vi "Set Path.vi"(8 "error in (no error)":errorcluster, 10 "Path":string, 11 "URI in":refnum<class "URI.lvclass">) -> (0 "error out":errorcluster, 3 "URI out":refnum<class "URI.lvclass">)   [LabVIEW 2020, in "URI.lvclass"]
uses:
  URI.lvclass
  URI.lvclass/URI.ctl
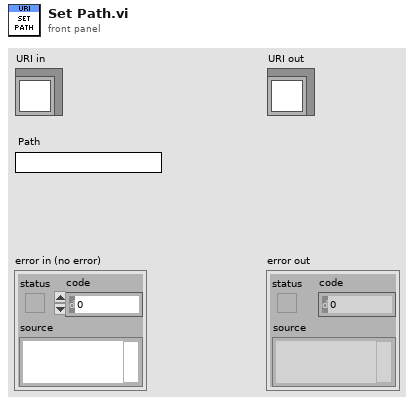
[diagram p1: front panel]
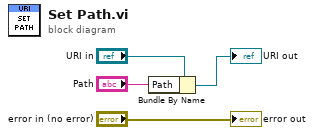
[diagram p0: block diagram]
diagram:
  n1 = Bundle By Name(cluster="URI in", "Path"="Path") -> (→"URI out":refnum<class "URI.lvclass">)
  "error out" <- "error in (no error)"
